vi "DHE_Getbpp.vi"() -> (7 "DHE_bpp":i32)   [LabVIEW 2016]
uses:
  private/vis/DHE_GBLDriverVariables.vi
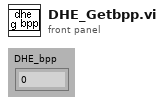
[diagram p1: front panel]
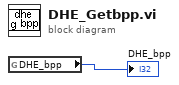
[diagram p0: block diagram]
diagram:
  n1 = global read "DHE_GBLDriverVariables.vi" "DHE_bpp"() -> (→"DHE_bpp":i32)
